vi "Add Relays.vi"(8 "error in (no error)":errorcluster, 11 "Node Ptr":u64 format="%.0x") -> (0 "error out":errorcluster)   [LabVIEW 2013, in "MUX Custom Device.lvlib"]
uses:
  MUX Custom Device.lvlib
  Relay Status.ctl
  Relay Data.ctl
  Switch.ctl
  <vilib>/NI Veristand/Custom Device API/Custom Device API.lvlib
  <vilib>/NI Veristand/Custom Device Tools/Custom Device Utility Library/Custom Device Utility Library.lvlib
panel:
  in  "Cancel":bool
  in  "OK":bool
  in  "Selected MUX Relays":T1[](array[typedef])
  in  "Available MUX Relays":T1[](array[typedef])
  in  "Tag":string
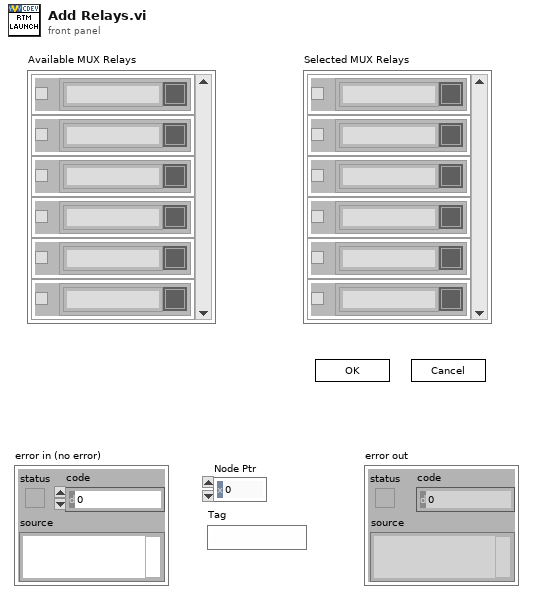
[diagram p1: front panel]
types:
  T1 = typedef "MUX Custom Device.lvlib/Relay Status.ctl" = cluster{"Present":bool, "Relay Data":T2}
  T2 = typedef "MUX Custom Device.lvlib/Relay Data.ctl" = cluster{"Relay Name":string, "State":T3}
  T3 = typedef "MUX Custom Device.lvlib/Switch.ctl" = bool
  T4 = cluster{"Available MUX Relays":refnum<vi>, "Selected MUX Relays":refnum<vi>}
  T5 = typedef "Custom Device API.lvlib/Custom Device Item Ref.ctl" = u64
  T6 = typedef "Relay Status.ctl" = cluster{"Present":bool, "Relay Data":T2}
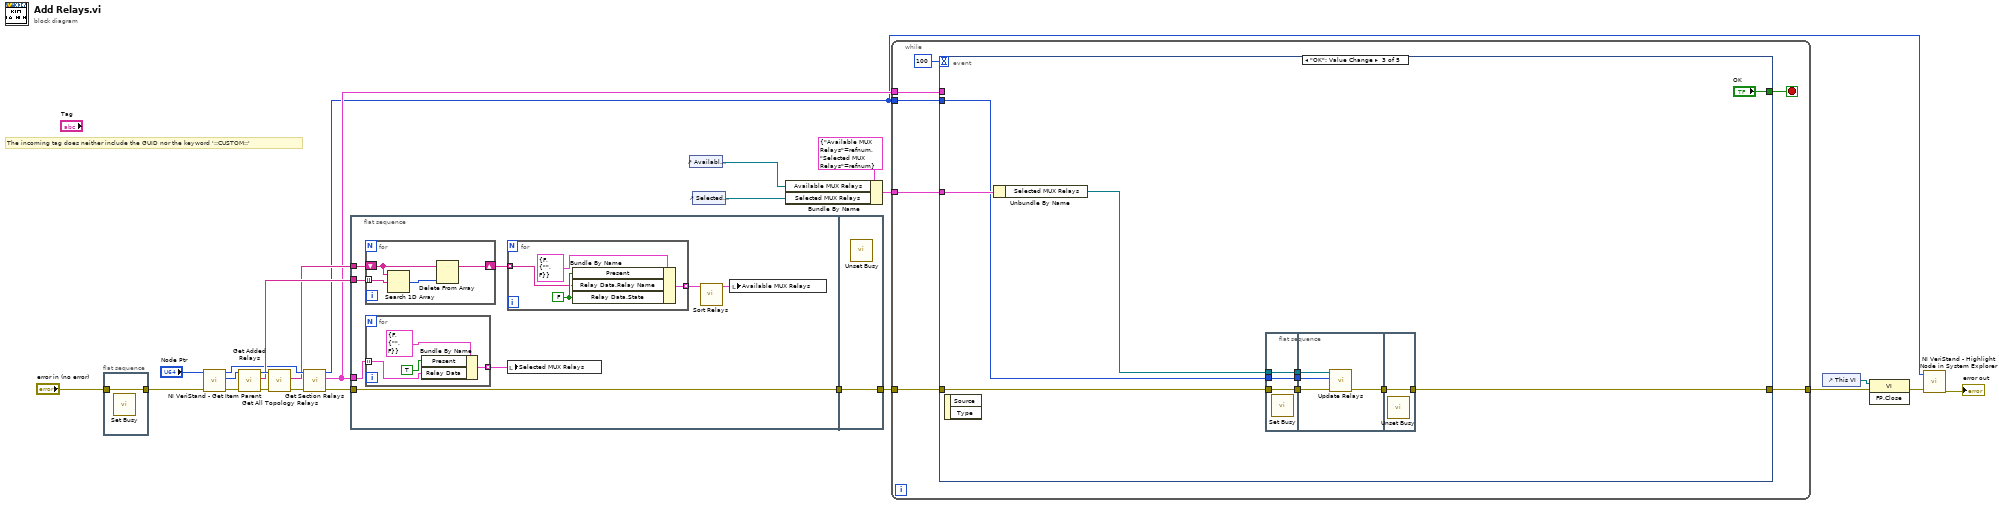
[diagram p0: block diagram]
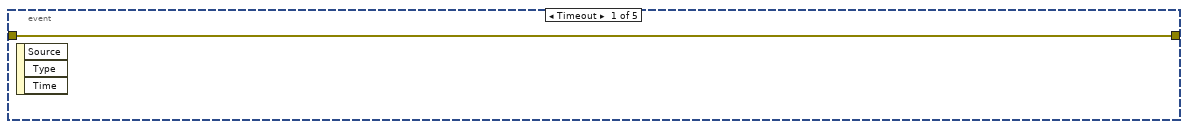
[diagram p2: hidden frame]
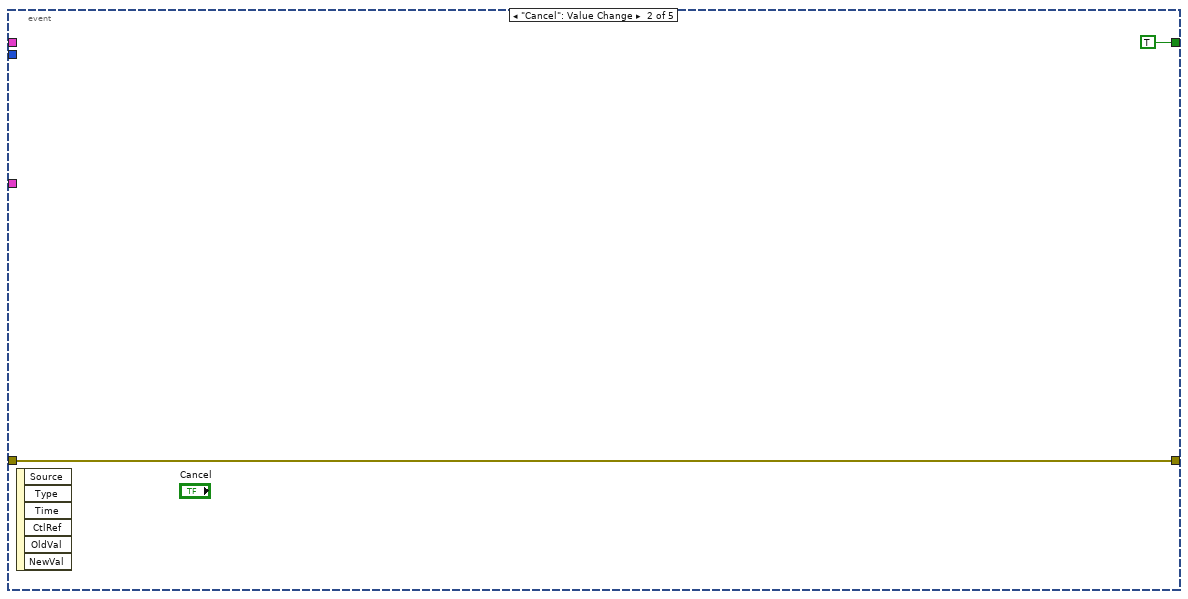
[diagram p3: hidden frame]
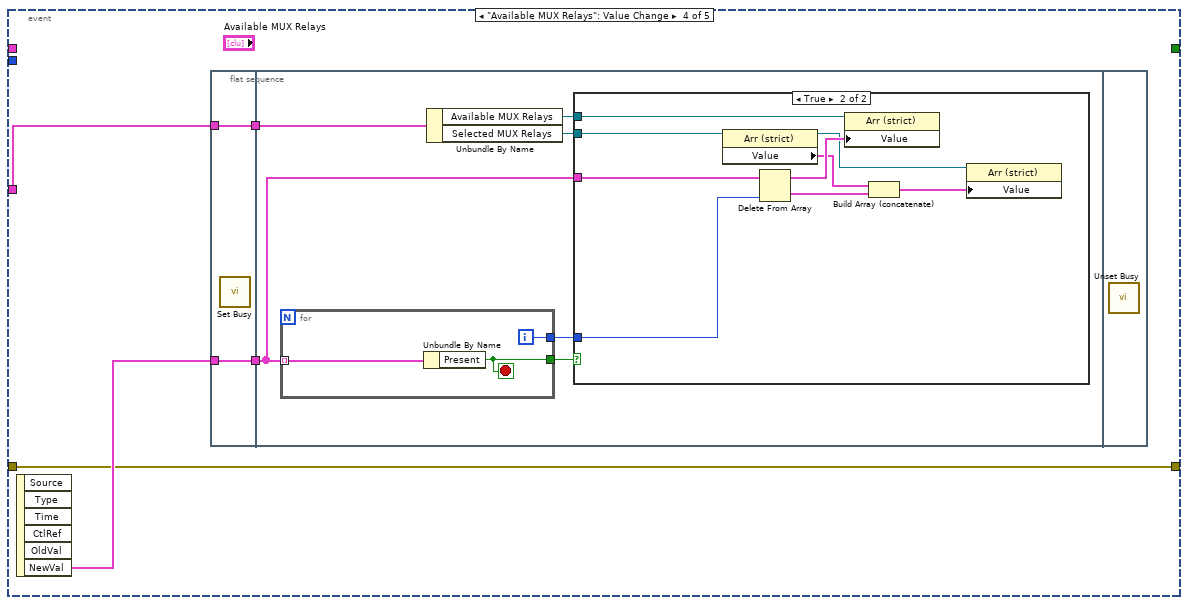
[diagram p4: hidden frame]
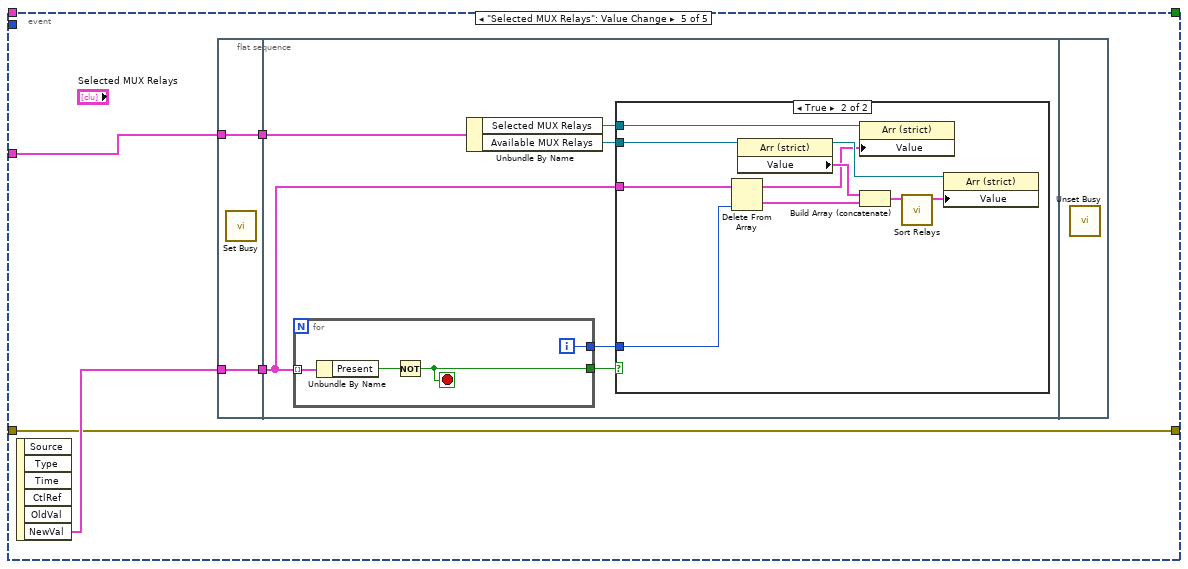
[diagram p6: hidden frame]
diagram:
  # "The incoming tag does neither include the GUID nor the keyword '::CUSTOM::'"
  n1 = flat-sequence {
    tunnel: "error in (no error)" -> [w25]
    tunnel: [w25] -> w14
    frame #0 {
      n2 = call <vilib>:"Set Busy.vi"() -> ()  [unwired: 10 in, 2 out]
    }
  }
  n3 = call <vilib>:"NI VeriStand - Get Item Parent.vi"("error in (no error)"=w14, "Item Ref in"="Node Ptr") -> ("error out"=w22:errorcluster, "Parent Ref"=w23:T5, "Item Ref out"=w17:T5)  [unwired: 6 in, 1 out]
  n4 = call "Get Added Relays.vi"("error in"=w22, "Custom Device Ref in"=w23) -> ("error out"=w21:errorcluster, "Added Relays Array"=w19:string[], "Custom Device Ref out"=w20:T5)  [unwired: 7 in]
  n5 = call "Get All Topology Relays.vi"("error in (no error)"=w21, "Custom Device Ref in"=w20) -> ("error out"=w18:errorcluster, "Available Relays"=w16:string[])  [unwired: 7 in, 1 out]
  n6 = call "Get Section Relays.vi"("error in (no error)"=w18, "MUX Section Ref in"=w17) -> ("error out"=w10:errorcluster, "Section Relays Array"=w6:T2[], "MUX Section Ref out"=w2:T5)  [unwired: 7 in]
  n7 = flat-sequence {
    tunnel: w19 -> [w33]
    tunnel: w16 -> [w32]
    tunnel: w6 -> [w30]
    tunnel: w10 -> [w28]
    tunnel: [w28] -> w9
    tunnel: [w46] -> w8
    tunnel: w9 -> [w46]
    frame #0 {
      n8 = for {
        tunnel: w33 -> [w45] mode=indexing
        shift-right: [w42] -> w31
        shift-left: w32 -> [w44]
        n9 = Search 1D Array(1D array=w44, element=w45) -> (index of element=w43:i32)  [unwired: 1 in]
        n10 = Delete From Array(array=w44, index=w43) -> (array with subset deleted=w42:string[])  [unwired: 1 in, 1 out]
      }
      n11 = for {
        tunnel: w30 -> [w34] mode=indexing
        tunnel: [w35] -> w29 mode=indexing
        n12 = Bundle By Name(cluster=T1 {"Present"=FALSE, "Relay Data"={"Relay Name"="", "State"=FALSE}} ("Relay Status"), "Present"=TRUE, "Relay Data"=w34) -> (w35:T1)
      }
      n13 = for {
        tunnel: w31 -> [w39] mode=indexing
        tunnel: [w38] -> w27 mode=indexing
        w40 = FALSE ("Present")
        n14 = Bundle By Name(cluster=T1 {"Present"=FALSE, "Relay Data"={"Relay Name"="", "State"=FALSE}} ("Relay Status"), "Present"=w40, "Relay Data.Relay Name"=w39, "Relay Data.State"=w40) -> (w38:T1)
      }
      n15 = local write "Selected MUX Relays"(w29) -> ()
      n16 = call "Sort Relays.vi"("Relays"=w27) -> ("Sorted Relays"=w26:T1[])  [unwired: 10 in]
      n17 = local write "Available MUX Relays"(w26) -> ()
    }
    frame #1 {
      n18 = call <vilib>:"Unset Busy.vi"() -> ()  [unwired: 11 in, 1 out]
    }
  }
  n19 = control-ref of="Available MUX Relays"() -> (w13:refnum<vi>)
  n20 = control-ref of="Selected MUX Relays"() -> (w12:refnum<vi>)
  n21 = Bundle By Name(cluster=T4 {"Available MUX Relays"=refnum, "Selected MUX Relays"=refnum} ("input cluster"), "Available MUX Relays"=w13, "Selected MUX Relays"=w12) -> (w7:T4)
  n22 = while {
    tunnel: w8 -> [w50]
    tunnel: w7 -> [w51]
    tunnel: w2 -> [w49]
    tunnel: w6 -> [w48]
    tunnel: [w47] -> w5
    stop <- w52 stop-if-true
    n23 = event shown="[2] \"OK\": Value Change" {
      selector: _ -> [_ _ _ _ _]
      dyn-events: _ -> [_ _ _ _ _]
      timeout: 100 -> [_ _ _ _ _]
      tunnel: [_ TRUE ("Stop") "OK" _ _] -> w52
      tunnel: w51 -> [_ _ w66 w78 w103]
      tunnel: w50 -> [w54 w55 w65 w77 w102]
      tunnel: w49 -> [_ _ w64 _ _]
      tunnel: w48 -> [_ _ _ _ _]
      tunnel: [w54 w55 w61 w77 w102] -> w47
      event Timeout {
        n24 = event-data() -> ()  [unwired: 1 in, 3 out]
      }
      event "Cancel": Value Change {
        n25 = event-data() -> ()  [unwired: 1 in, 6 out]
      }
      event "OK": Value Change {
        n26 = event-data() -> ()  [unwired: 1 in, 2 out]
        n27 = Unbundle By Name(w66) -> ("Selected MUX Relays"=w63:refnum<vi>)
        n28 = flat-sequence {
          tunnel: w63 -> [w67]
          tunnel: w64 -> [w68]
          tunnel: w65 -> [w69]
          tunnel: [w69] -> w59
          tunnel: [w68] -> w58
          tunnel: [w67] -> w57
          tunnel: [w70] -> w60
          tunnel: w59 -> [w73]
          tunnel: w58 -> [w72]
          tunnel: w57 -> [w71]
          tunnel: [w74] -> w61
          tunnel: w60 -> [w74]
          frame #0 {
            n29 = call <vilib>:"Set Busy.vi"() -> ()  [unwired: 10 in, 2 out]
          }
          frame #1 {
            n30 = call "Update Relays.vi"("error in (no error)"=w73, "MUX Section Ref in"=w72, "Selected MUX Relays"=w71) -> ("error out"=w70:errorcluster)  [unwired: 8 in]
          }
          frame #2 {
            n31 = call <vilib>:"Unset Busy.vi"() -> ()  [unwired: 11 in, 1 out]
          }
        }
      }
      event "Available MUX Relays": Value Change {
        n32 = event-data() -> ("NewVal"=w79:T1[])  [unwired: 1 in, 5 out]
        n33 = flat-sequence {
          tunnel: w78 -> [w80]
          tunnel: w79 -> [w81]
          tunnel: [w81] -> w76
          tunnel: [w80] -> w75
          tunnel: w76 -> [w87]
          tunnel: w75 -> [w85]
          frame #0 {
            n34 = call <vilib>:"Set Busy.vi"() -> ()  [unwired: 10 in, 2 out]
          }
          frame #1 {
            n35 = for {
              tunnel: w87 -> [w99] mode=indexing
              tunnel: [w98] -> w86
              tunnel: [w97] -> w82
              i -> [w98]
              stop <- w97 stop-if-true
              n36 = Unbundle By Name(w99) -> ("Present"=w97:bool)
            }
            n37 = Unbundle By Name(w85) -> ("Available MUX Relays"=w84:refnum<vi>, "Selected MUX Relays"=w83:refnum<vi>)
            n38 = case shown="True" w82 {
              tunnel: w87 -> [_ w96]
              tunnel: w86 -> [_ w95]
              tunnel: w84 -> [_ w93]
              tunnel: w83 -> [_ w91]
              frame False {
              }
              frame True {
                n39 = property class="Arr (strict)"(reference=w91) -> (reference out=w88:refnum<vi>, "Value"=w90:T6[])  [unwired: 1 in, 1 out]
                n40 = Delete From Array(array=w96, index=w95) -> (deleted portion=w94:T1, array with subset deleted=w92:T1[])  [unwired: 1 in]
                n41 = property class="Arr (strict)"(reference=w93, "Value"=w92) -> ()  [unwired: 1 in, 2 out]
                n42 = Build Array (concatenate)(w90, w94) -> (w89:T1[])
                n43 = property class="Arr (strict)"(reference=w88, "Value"=w89) -> ()  [unwired: 1 in, 2 out]
              }
            }
          }
          frame #2 {
            n44 = call <vilib>:"Unset Busy.vi"() -> ()  [unwired: 11 in, 1 out]
          }
        }
      }
      event "Selected MUX Relays": Value Change {
        n45 = event-data() -> ("NewVal"=w104:T1[])  [unwired: 1 in, 5 out]
        n46 = flat-sequence {
          tunnel: w103 -> [w105]
          tunnel: w104 -> [w106]
          tunnel: [w106] -> w101
          tunnel: [w105] -> w100
          tunnel: w101 -> [w112]
          tunnel: w100 -> [w108]
          frame #0 {
            n47 = call <vilib>:"Set Busy.vi"() -> ()  [unwired: 10 in, 2 out]
          }
          frame #1 {
            n48 = for {
              tunnel: w112 -> [w126] mode=indexing
              tunnel: [w124] -> w111
              tunnel: [w123] -> w107
              i -> [w124]
              stop <- w123 stop-if-true
              n49 = Unbundle By Name(w126) -> ("Present"=w125:bool)
              n50 = Not(x=w125) -> (.not. x?=w123:bool)
            }
            n51 = Unbundle By Name(w108) -> ("Selected MUX Relays"=w110:refnum<vi>, "Available MUX Relays"=w109:refnum<vi>)
            n52 = case shown="True" w107 {
              tunnel: w112 -> [_ w122]
              tunnel: w111 -> [_ w121]
              tunnel: w110 -> [_ w120]
              tunnel: w109 -> [_ w119]
              frame False {
              }
              frame True {
                n53 = Delete From Array(array=w122, index=w121) -> (deleted portion=w115:T1, array with subset deleted=w116:T1[])  [unwired: 1 in]
                n54 = property class="Arr (strict)"(reference=w119) -> (reference out=w117:refnum<vi>, "Value"=w118:T6[])  [unwired: 1 in, 1 out]
                n55 = property class="Arr (strict)"(reference=w120, "Value"=w116) -> ()  [unwired: 1 in, 2 out]
                n56 = Build Array (concatenate)(w118, w115) -> (w114:T1[])
                n57 = call "Sort Relays.vi"("Relays"=w114) -> ("Sorted Relays"=w113:T1[])  [unwired: 10 in]
                n58 = property class="Arr (strict)"(reference=w117, "Value"=w113) -> ()  [unwired: 1 in, 2 out]
              }
            }
          }
          frame #2 {
            n59 = call <vilib>:"Unset Busy.vi"() -> ()  [unwired: 11 in, 1 out]
          }
        }
      }
    }
  }
  n60 = control-ref of="This VI"() -> (w4:refnum<vi>)
  n61 = invoke class="VI" method="FP.Close"(reference=w4, error in=w5) -> (error out=w3:errorcluster)  [unwired: 1 in, 2 out]
  n62 = call <vilib>:"NI VeriStand - Highlight Node in System Explorer.vi"("error in (no error)"=w3, "Item Ref in"=w2) -> ("error out"=→"error out":errorcluster)  [unwired: 8 in, 1 out]
